vi "Write Data.vi"(8 "error in (no error)":errorcluster, 10 "Data":string, 11 "Missing Plugin configuration in":refnum<class "Missing Plugin configuration.lvclass">) -> (0 "error out":errorcluster, 3 "Missing Plugin configuration out":refnum<class "Missing Plugin configuration.lvclass">)   [LabVIEW 2014, in "Missing Plugin configuration.lvclass"]
uses:
  Missing Plugin configuration.lvclass
  Missing Plugin configuration.lvclass/Missing Plugin configuration.ctl
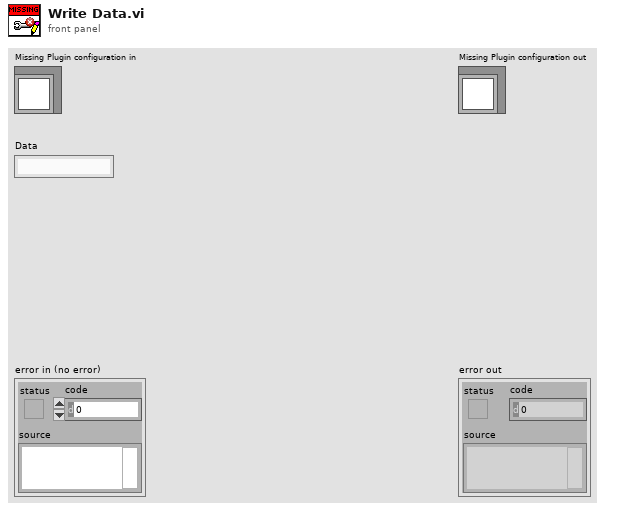
[diagram p1: front panel]
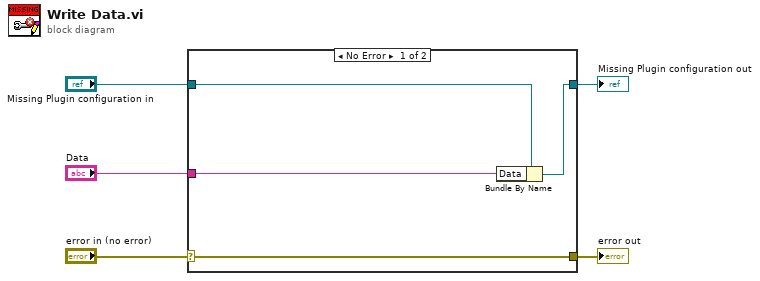
[diagram p0: block diagram]
diagram:
  n1 = case shown="No Error" "error in (no error)" {
    selector: "error in (no error)" -> [w9 w10]
    tunnel: [w9 w10] -> w4
    tunnel: [w7 w11] -> w2
    tunnel: "Missing Plugin configuration in" -> [w8 w11]
    tunnel: "Data" -> [w6 _]
    frame No Error {
      n2 = Bundle By Name(cluster=w8, "Data"=w6) -> (w7:refnum<class "Missing Plugin configuration.lvclass">)
    }
    frame Error {
    }
  }
  "error out" <- w4
  "Missing Plugin configuration out" <- w2
